vi "delete EIP tag.vi"(8 "error in":errorcluster, 9 "Tag Name":string, 10 "Network Path":string, 11 "EIP Tags configuration in":refnum<class "EIP Tags Configuration.lvclass">) -> (0 "error out":errorcluster, 3 "EIP Tags configuration out":refnum<class "EIP Tags Configuration.lvclass">)   [LabVIEW 2013, in "EIP Tags Configuration.lvclass"]
uses:
  EIP Tags Configuration.lvclass
  EIP Tags Configuration.lvclass/EIP Tags Configuration.ctl
  <vilib>/NI/Tag Bus Module Framework/root configuration/TBM configuration.lvclass
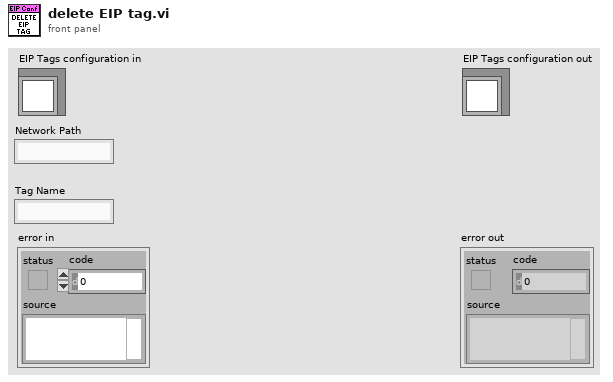
[diagram p1: front panel]
types:
  T1 = typedef "EIP Tags Configuration.lvclass/eip tag definition.ctl" = cluster{"eip tag types":T2, "unique tag name":string, "Number of Elements":u32}
  T2 = typedef "EIP Tags Configuration.lvclass/eip tag types.ctl" = enum16{"SINT", "INT", "DINT", "REAL", "BOOL", "STRING"}
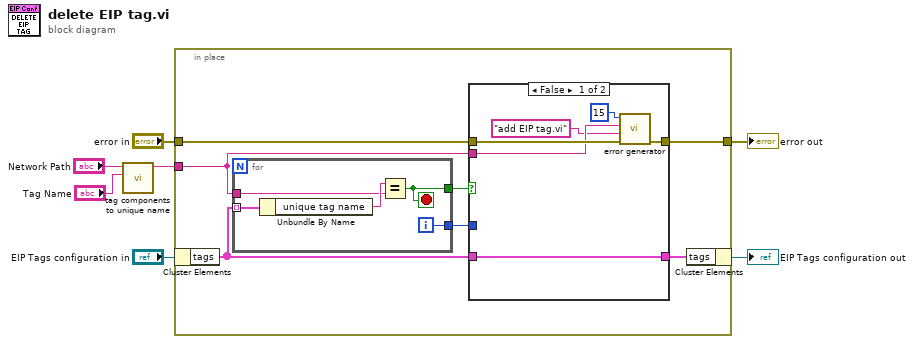
[diagram p0: block diagram]
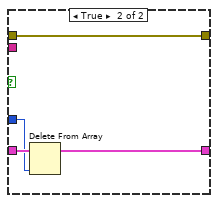
[diagram p2: hidden frame]
diagram:
  n1 = call "tag components to unique name.vi"("Tag Name"="Tag Name", "Network Path"="Network Path") -> ("unique name"=w2:string)  [unwired: 9 in]
  n2 = in-place {
    in-place-border: "error in" -> [w12]
    in-place-border: w2 -> [w9]
    in-place-border: [w13] -> w1
    n3 = in-place-cluster #1("EIP Tags configuration in") -> ("tags"=w10:T1[])
    n4 = for {
      tunnel: w10 -> [w29] mode=indexing
      tunnel: w9 -> [w27]
      tunnel: [w26] -> w14
      tunnel: [w25] -> w8
      i -> [w25]
      stop <- w26 stop-if-true
      n5 = Unbundle By Name(w29) -> ("unique tag name"=w28:string)
      n6 = Equal?(x=w28, y=w27) -> (x = y?=w26:bool)
    }
    n7 = case shown="False" w14 {
      tunnel: [w20 w24] -> w13
      tunnel: w12 -> [w19 w24]
      tunnel: [w17 w22] -> w11
      tunnel: w10 -> [w17 w23]
      tunnel: w9 -> [w16 _]
      tunnel: w8 -> [_ w21]
      frame False {
        n8 = call <vilib>:"error generator.vi"("error in"=w19, "source"="add EIP tag.vi", "append error message"=w16, "error code (0)"=15) -> ("error out"=w20:errorcluster)  [unwired: 7 in]
      }
      frame True {
        n9 = Delete From Array(array=w23, index=w21) -> (array with subset deleted=w22:T1[])  [unwired: 1 in, 1 out]
      }
    }
    n10 = in-place-cluster #1("tags"=w11) -> (→"EIP Tags configuration out":refnum<class "EIP Tags Configuration.lvclass">)
  }
  "error out" <- w1
